vi "Posicionador_VF_Para_Desarrollador.vi"() -> ()   [LabVIEW 2015]
uses:
  <vilib>/Instr/_visa.llb/VISA Configure Serial Port (Instr).vi
panel:
  out "Caracterización Terminada":bool
  in  "Puerto Serial del Gaussmetro":refnum<visa-resource-name>="COM5"
  in  "Ruta de archivo de medición":path=path "C:/Users/PIV/Desktop/Enrico/prueba1.txt"
  out "Medición de campo magnético \nen Teslas [T]":string
  out "?":string="mm"
  out "?":string="mm"
  in  "Listo Y":bool
  in  "Listo X":bool
  in  "Abajo":bool
  in  "Arriba":bool
  in  "Derecha":bool
  in  "Izquierda":bool
  out "Posiciòn en eje X":i32
  out "Posiciòn en eje Y":i32
  in  "Longitud del imán":i32
  in  "Altura del imán":i32
  in  "Puerto Serial de Arduino":refnum<visa-resource-name>="COM12"
  # "Los archivos ejecutables para este programa se encuentran en el repositorio https://github.com/SebRey1995/Posicionador_Caracterizacion.git \n\nPARA LA SECCIÓN DE IDE DE ARDUINO: El archivo denominado \"motor2.ino\" se encuentra en la carpeta denominada \"motor2\". \nPARA LA SECCIÓN DEL EJECUTABLE: El archivo denominado \"Posicionador_VF.exe\" se encuentra en la carpeta \"LabVIEW\".\n\nNota: Para conexión serial entre Gaussmetro y PC, será necesario instalar el archivo ejecutable contenido en la raíz del repositorio proporcionado al principio de este manual. El nombre del archivo es PL2303_64bit_Installer.exe. \nENCENDER GAUSSMETRO MODELO 6010\nIDE DE ARDUINO\n1.  Los pines para la conexión del driver del motor con el Arduino están indicados en el archivo \"motor2.ino\" mediante las variables \"DirPin\", \"StepPin\", \"EnnablePin\" para el motor en X, y \"DirPin2\", \"StepPin2\", \"EnnablePin2\", para el motor en Y. El primer pin refiere a la Dirección; el segundo es el pin para mandarle el tren de pulsos y el tercero para habilitar el motor.\n2.  Para modificar el desplazamiento de 1mm de ambos motores, se deberá modificar el archivo \"motor2.ino\" en la sección después del loop denominada \"void stepMotor\" y \"void Stepmotor2, modificar la variable steps por la cantidad de desplazamiento deseado, tomando en cuenta que steps = 1000 = 1mm de desplazamiento.\n\nAbrir PROGRAMA Posicionador_VF.exe  con los archivos .aliases y .ini en la misma carpeta en la que se ejecuta el archivo  Posicionador_VF.exe \n3.  En el apartado \"Puerto Serial de Arduino\" en la parte superior izquierda, indicar el puerto serial del Arduino. Para verificar en qué puerto se localiza, dirigirse al menú inicio y escribir \"Administrador de dispositivos\". Seguido de esto se dará clic en la opción con el mismo nombre y, en la ventana que emerge, se buscará el apartado \"Puertos COM y LPT\". El puerto del Arduino lleva por nombre inicial \"Arduino\".\n4.  Para seleccionar el puerto del Gaussmetro, dirigirse como en el paso anterior al Administrador de dispositivos y en el apartado Puerto COM y LPT buscar el nombre \"Prolific USB-to-Serial Comm Port\", y el nombre del puerto se especificará entre paréntesis. Este nombre de puerto se especificará en el apartado \"Puerto Serial del Gaussmetro\" ubicado debajo del apartado \"Puerto Serial de Arduino\". \n5.  Ingresar la longitud [en mm] del imán.\n6.  Ingresar la altura [en mm] del imán\n7.  Crear un archivo de texto .txt en la computadora (ubicación a elección) para guardar archivos \n8.  En el apartado \"Ruta de archivo de medición\" se deberá introducir la ubicación del archivo creado en el paso anterior.\n9.  Colocar el imán a caracterizar de forma que la probeta se encuentre del lado superior izquierdo de este. Esto debido a que el movimiento horizontal es hacia la derecha, y el movimiento vertical es hacia abajo.\n10. Verificar Conexión entre el Arduino y el posicionador. Esto se realiza observando un foco led color naranja en la carcasa del motor negro ubicado en el extremo izquierdo del riel horizontal (esto indica que la comunicación serial fue exitosa).\n11.  En caso de estar apagada la luz led naranja del motor, se deberá reiniciar el programa. Para esto se presionará el botón rojo de la parte superior izquierda y se esperará unos segundos hasta ver la luz LED naranja encenderse. Una vez encendida esta luz, se correrá el programa con la flecha blanca de la parte superior izquierda.\n12.  Se deberá iniciar colocando la posición inicial en X (Derecha e Izquierda). Una vez finalizada la posición inicial en X, oprimir el botón \"Listo X\". Al finalizar, deberá parpadear una vez el foco led naranja y se volverá a encender.\n13.  Seguido, se colocará la posición inicial en Y (Arriba y Abajo). Una vez finalizada la posición inicial en Y, oprimir el botón \"Listo Y\". Al finalizar esto, parpadeará una vez el LED naranja y se dará inicio la caracterización deseada.\n\nNOTA: SÓLO PARA LA POSICIÓN DE INICIO EN LA QUE POSICIÓN X = 0 Y POSICIÓN Y = 0, SE TOMARÁ LA MEDICIÓN DE ESE PUNTO, PERO NO SE DESPLAZARÁ 1mm A LA DERECHA. PARA TODOS LOS DEMÁS CASOS SÍ SE DESPLAZARÁ NORMALMENTE.\n\nCreado por:\nSebastian A. Reyes Romero\nContacto: rerosa@ier.unam.mx"
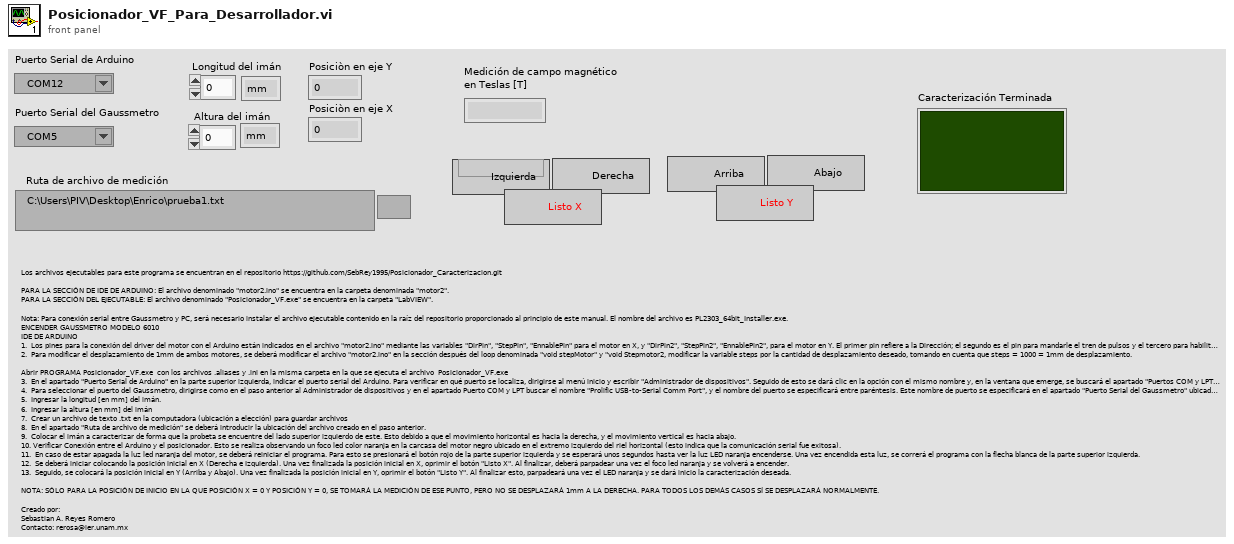
[diagram p1: front panel]
types:
  T1 = enum16{"open", "open or create", "create or replace", "create", "open (read only)"}
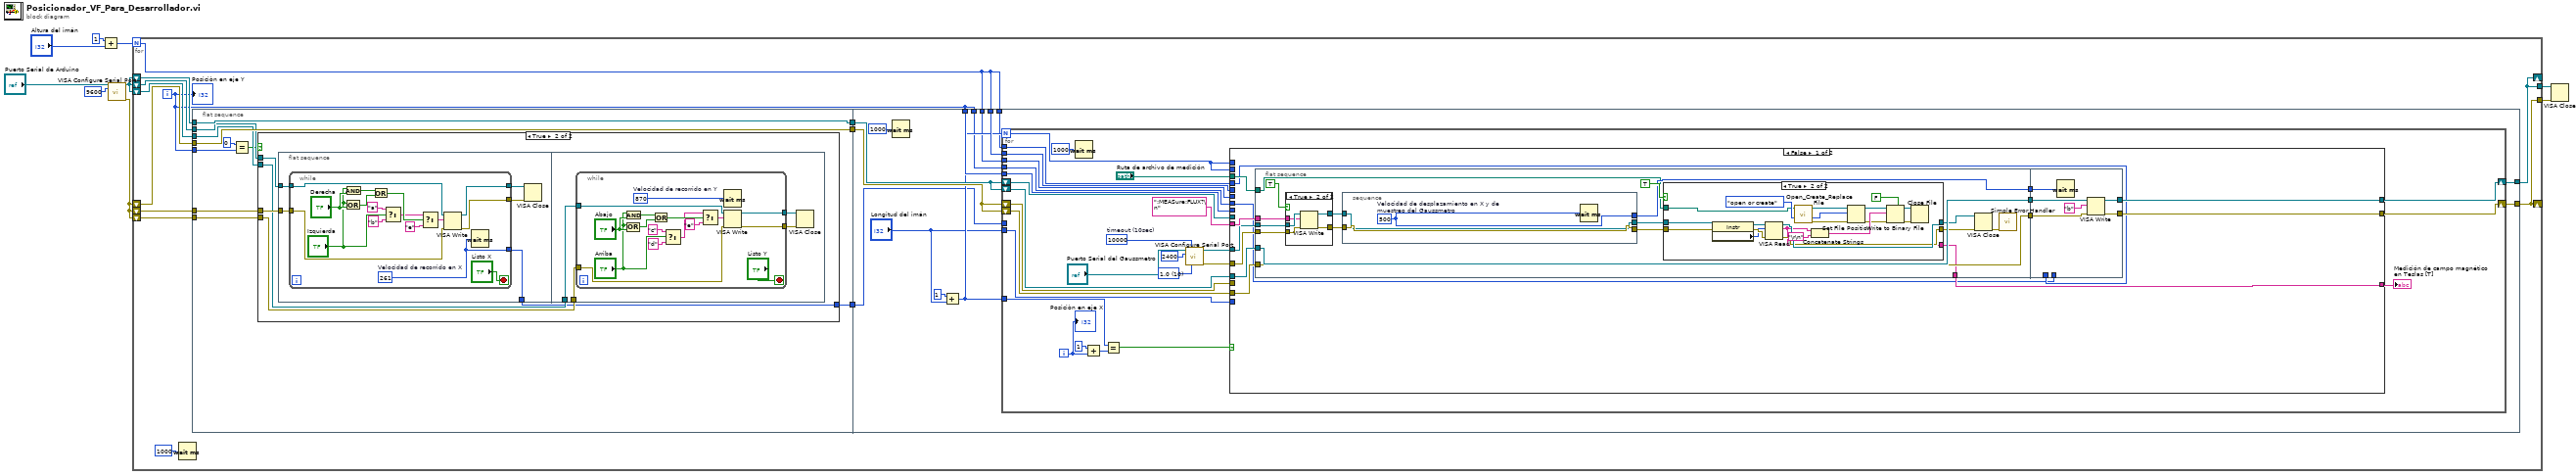
[diagram p0: block diagram]
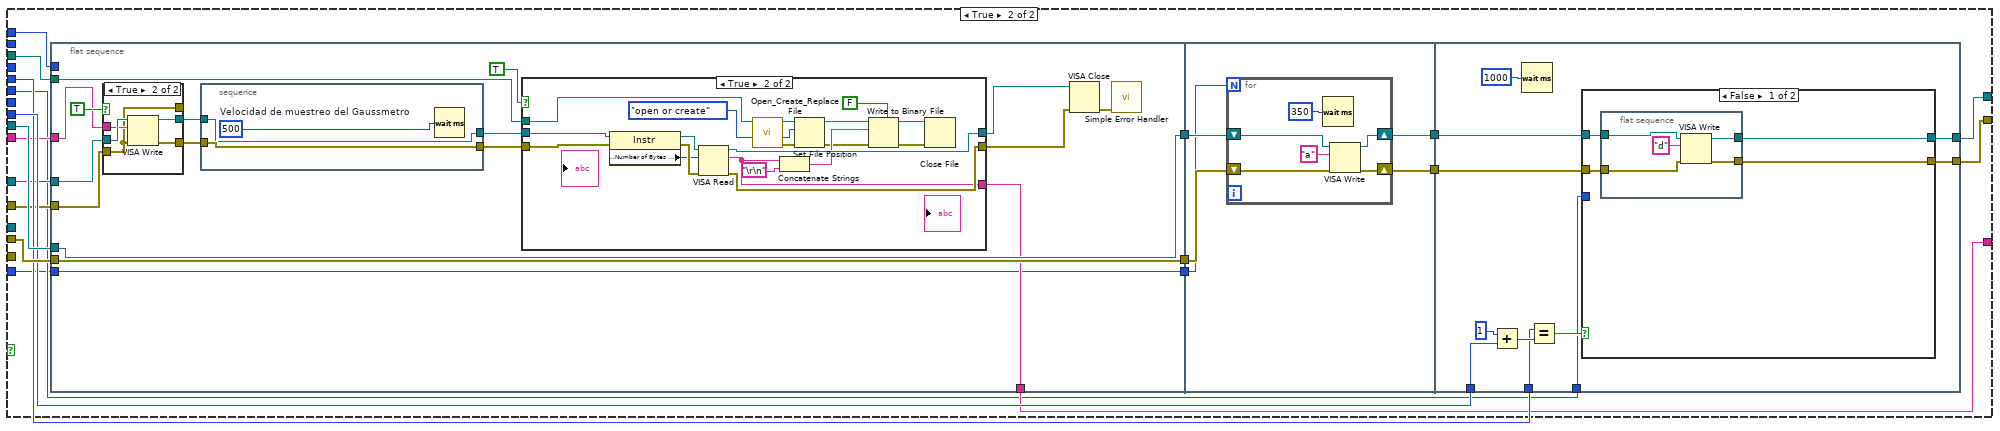
[diagram p5: hidden frame]
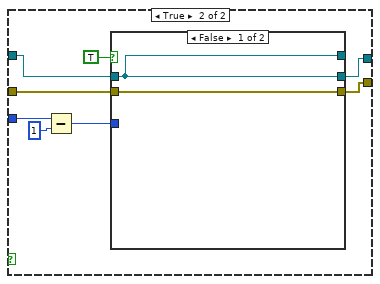
[diagram p8: hidden frame]
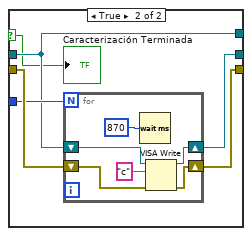
[diagram p9: hidden frame]
diagram:
  n1 = Add(x=1, y="Altura del imán") -> (x+y=w5:i32)
  n2 = call-poly "VISA Configure Serial Port"("VISA resource name"="Puerto Serial de Arduino", "baud rate (9600)"=u32 9600) -> ("VISA resource name out"=w3:refnum<visa-resource-name>, "error out"=w4:errorcluster)  [unwired: 12 in]
  n3 = for {
    N: w5 -> [w11]
    shift-right: [w13] -> _
    shift-right: [w14] -> _
    shift-left: w4 -> [w23]
    shift-left: w3 -> [w19]
    shift-left: w4 -> [w18]
    shift-left: w4 -> [w17]
    shift-left: w3 -> [w15]
    shift-left: w3 -> [w16]
    tunnel: [w14] -> w2
    tunnel: [w13] -> w1
    i -> [w12]
    n4 = Wait (ms)(milliseconds to wait=u32 1000) -> ()  [unwired: 1 out]
    n5 = flat-sequence {
      tunnel: w23 -> [w33]
      tunnel: [w30] -> w21
      tunnel: [w33] -> w20
      tunnel: w19 -> [w29]
      tunnel: w18 -> [w32]
      tunnel: w17 -> [w31]
      tunnel: w16 -> [w30]
      tunnel: w15 -> [w28]
      tunnel: w12 -> [w27]
      tunnel: [w24] -> w10
      tunnel: [w92] -> w14
      tunnel: [w93] -> w13
      tunnel: w12 -> [w89]
      tunnel: w11 -> [w88]
      tunnel: w21 -> [w91]
      tunnel: w20 -> [w90]
      tunnel: w11 -> [w84]
      tunnel: w12 -> [w83]
      tunnel: w11 -> [w82]
      tunnel: w10 -> [w81]
      frame #0 {
        n6 = Equal?(x=0, y=w27) -> (x = y?=w25:bool)
        n7 = case shown="True" w25 {
          tunnel: w32 -> [_ w38]
          tunnel: w31 -> [_ w37]
          tunnel: w29 -> [_ w36]
          tunnel: w28 -> [_ w35]
          tunnel: [_ w34] -> w24
          frame False {
          }
          frame True {
            n8 = flat-sequence {
              tunnel: w35 -> [w43]
              tunnel: w38 -> [w42]
              tunnel: [w39] -> w34
              tunnel: w36 -> [w63]
              tunnel: w37 -> [w62]
              frame #0 {
                n9 = while {
                  tunnel: w43 -> [w50]
                  tunnel: w42 -> [w49]
                  tunnel: [w46] -> w41
                  tunnel: [w45] -> w40
                  tunnel: [w44] -> w39
                  stop <- "Listo X" stop-if-true
                  w44 = u32 261  # Velocidad de recorrido en X
                  n10 = Or(x="Izquierda", y="Derecha") -> (x .or. y?=w56:bool)
                  n11 = And(x="Izquierda", y="Derecha") -> (x .and. y?=w58:bool)
                  n12 = Or(x=w58, y=w56) -> (x .or. y?=w55:bool)
                  n13 = Select(t="a", s="Izquierda", f="b") -> (s? t:f=w48:string)
                  n14 = Select(t=w48, s=w55, f="e") -> (s? t:f=w51:string)
                  n15 = VISA Write(VISA resource name=w50, write buffer=w51, error in (no error)=w49) -> (VISA resource name out=w45:refnum<visa-resource-name>, error out=w46:errorcluster)  [unwired: 1 out]
                  n16 = Wait (ms)(milliseconds to wait=w44) -> ()  [unwired: 1 out]
                }
                n17 = VISA Close(VISA resource name=w40, error in (no error)=w41) -> ()  [unwired: 1 out]
              }
              frame #1 {
                n18 = while {
                  tunnel: w63 -> [w70]
                  tunnel: w62 -> [w69]
                  tunnel: [w65] -> w61
                  tunnel: [w64] -> w60
                  stop <- "Listo Y" stop-if-true
                  w66 = u32 870  # Velocidad de recorrido en Y
                  n19 = Or(x="Arriba", y="Abajo") -> (x .or. y?=w77:bool)
                  n20 = And(x="Arriba", y="Abajo") -> (x .and. y?=w78:bool)
                  n21 = Or(x=w78, y=w77) -> (x .or. y?=w76:bool)
                  n22 = Select(t="c", s="Arriba", f="d") -> (s? t:f=w67:string)
                  n23 = Select(t=w67, s=w76, f="e") -> (s? t:f=w71:string)
                  n24 = Wait (ms)(milliseconds to wait=w66) -> ()  [unwired: 1 out]
                  n25 = VISA Write(VISA resource name=w70, write buffer=w71, error in (no error)=w69) -> (VISA resource name out=w64:refnum<visa-resource-name>, error out=w65:errorcluster)  [unwired: 1 out]
                }
                n26 = VISA Close(VISA resource name=w60, error in (no error)=w61) -> ()  [unwired: 1 out]
              }
            }
          }
        }
      }
      frame #1 {
        n27 = Wait (ms)(milliseconds to wait=u32 1000) -> ()  [unwired: 1 out]
        n28 = Add(x=1, y="Longitud del imán") -> (x+y=w86:i32)
        n29 = for {
          N: w86 -> [w115]
          shift-right: [w118] -> w93
          shift-left: w91 -> [w120]
          shift-right: [w117] -> w92
          shift-left: w90 -> [w119]
          shift-left: w91 -> [w116]
          shift-left: w90 -> [w114]
          tunnel: w86 -> [w110]
          tunnel: w89 -> [w109]
          tunnel: w88 -> [w108]
          tunnel: w84 -> [w97]
          tunnel: w83 -> [w96]
          tunnel: w82 -> [w95]
          tunnel: w81 -> [_]
          tunnel: "Longitud del imán" -> [w94]
          i -> [w113]
          w100 = u16 10 items=["1.0"=10, "1.5"=15, "2.0"=20] ("stop bits (10: 1 bit)")
          w103 = u32 10000  # timeout (10sec)
          n30 = Wait (ms)(milliseconds to wait=u32 1000) -> ()  [unwired: 1 out]
          n31 = Add(x=1, y=w113) -> (x+y=w111:i32)
          n32 = Equal?(x=w110, y=w111) -> (x = y?=w121:bool)
          n33 = call-poly "VISA Configure Serial Port"("VISA resource name"="Puerto Serial del Gaussmetro", "timeout (10sec)"=w103, "baud rate (9600)"=u32 2400, "stop bits (10: 1 bit)"=w100) -> ("VISA resource name out"=w99:refnum<visa-resource-name>, "error out"=w98:errorcluster)  [unwired: 5 in, 5 out]
          n34 = case shown="False" w121 {
            tunnel: w120 -> [_ w209]
            tunnel: w119 -> [_ w208]
            tunnel: [w133 w207] -> w118
            tunnel: [w132 w206] -> w117
            tunnel: w115 -> [_ w205]
            tunnel: w116 -> [w135 _]
            tunnel: w114 -> [w134 _]
            tunnel: w115 -> [_ _]
            tunnel: w109 -> [_ w202]
            tunnel: w108 -> [_ w201]
            tunnel: [w128 w198] -> w106
            tunnel: ":MEASure:FLUX?\n" ("Dato de entrada para\nobtención de flujo magnético 2") -> [w127 w197]
            tunnel: "Ruta de archivo de medición" -> [w126 w196]
            tunnel: w99 -> [w125 w195]
            tunnel: w98 -> [w124 w194]
            tunnel: w97 -> [w123 _]
            tunnel: w96 -> [w122 _]
            tunnel: w95 -> [_ w193]
            tunnel: w94 -> [_ w191]
            frame False {
              n35 = flat-sequence {
                tunnel: w134 -> [w151]
                tunnel: w135 -> [w152]
                tunnel: [w152] -> w131
                tunnel: [w151] -> w130
                tunnel: [w141] -> w129
                tunnel: [w140] -> w128
                tunnel: w127 -> [w139]
                tunnel: w126 -> [w138]
                tunnel: w125 -> [w137]
                tunnel: w124 -> [w136]
                tunnel: [w189] -> w132
                tunnel: [w190] -> w133
                tunnel: w123 -> [_]
                tunnel: w122 -> [_]
                tunnel: w129 -> [w185]
                tunnel: w130 -> [w187]
                tunnel: w131 -> [w188]
                frame #0 {
                  n36 = case shown="True" TRUE ("write") {
                    tunnel: [w157 w162] -> w145
                    tunnel: w137 -> [w156 w161]
                    tunnel: w136 -> [w157 w160]
                    tunnel: [w156 w159] -> w143
                    tunnel: w139 -> [_ w158]
                    frame False {
                    }
                    frame True {
                      n37 = VISA Write(VISA resource name=w161, write buffer=w158, error in (no error)=w160) -> (VISA resource name out=w159:refnum<visa-resource-name>, error out=w162:errorcluster)  [unwired: 1 out]
                    }
                  }
                  n38 = stacked-sequence {
                    tunnel: w145 -> [w155]
                    tunnel: [w155] -> w144
                    tunnel: w143 -> [w154]
                    tunnel: [w154] -> w142
                    tunnel: [w153] -> w141
                    frame #0 {
                      w153 = u32 500  # Velocidad de desplazamiento en X y de muestreo del Gaussmetro
                      n39 = Wait (ms)(milliseconds to wait=w153) -> ()  [unwired: 1 out]
                    }
                  }
                  n40 = case shown="True" TRUE ("read") {
                    tunnel: w144 -> [w164 w181]
                    tunnel: [w164 w178] -> w149
                    tunnel: [w163 w184] -> w148
                    tunnel: w142 -> [w163 w183]
                    tunnel: [_ w166] -> w140
                    tunnel: w138 -> [_ w165]
                    frame False {
                    }
                    frame True {
                      n41 = property class="Instr"(reference=w183, error in=w181) -> (reference out=w182:refnum<visa-resource-name>, error out=w180:errorcluster, "Serial Settings:Number of Bytes at Serial Port"=w179:u32)
                      n42 = VISA Read(VISA resource name=w182, byte count=w179, error in (no error)=w180) -> (VISA resource name out=w184:refnum<visa-resource-name>, read buffer=w166:string, error out=w178:errorcluster)  [unwired: 1 out]
                      n43 = call <vilib>:"Open_Create_Replace File.vi"("function (open:0)"=T1."open or create", "file path"=w165) -> ("error out"=w176:errorcluster, "file size (bytes)"=w174:i32, "refnum"=w175:refnum<file>)  [unwired: 6 in, 1 out]
                      n44 = Concatenate Strings(w166, "\r\n") -> (w170:string)
                      n45 = Set File Position(offset (in bytes) (0)=w174, refnum=w175, error in=w176) -> (refnum out=w169:refnum<file>, error out=w168:errorcluster)  [unwired: 1 in]
                      n46 = Write to Binary File(file (use dialog)=w169, data=w170, error in=w168, 5:FALSE ("prepend array or string size? (T)")) -> (refnum out=w172:refnum<file>, error out=w173:errorcluster)  [unwired: 2 in, 1 out]
                      n47 = Close File(refnum=w172, error in=w173) -> ()  [unwired: 2 out]
                    }
                  }
                  n48 = VISA Close(VISA resource name=w148, error in (no error)=w149) -> (error out=w147:errorcluster)
                  n49 = call <vilib>:"Simple Error Handler.vi"("error in (no error)"=w147) -> ()  [unwired: 1 in, 8 out]
                }
                frame #1 {
                  n50 = Wait (ms)(milliseconds to wait=w185) -> ()  [unwired: 1 out]
                  n51 = VISA Write(VISA resource name=w188, write buffer="b", error in (no error)=w187) -> (VISA resource name out=w190:refnum<visa-resource-name>, error out=w189:errorcluster)  [unwired: 1 out]
                }
              }
            }
            frame True {
              n52 = flat-sequence {
                tunnel: w205 -> [_]
                tunnel: w208 -> [w225]
                tunnel: w209 -> [w226]
                tunnel: [w226] -> w200
                tunnel: [w225] -> w199
                tunnel: [w215] -> w198
                tunnel: w197 -> [w214]
                tunnel: w196 -> [w213]
                tunnel: w195 -> [w212]
                tunnel: w194 -> [w211]
                tunnel: [w210] -> w192
                tunnel: w191 -> [w210]
                tunnel: [w261] -> w204
                tunnel: [w260] -> w203
                tunnel: w200 -> [w263]
                tunnel: w199 -> [w262]
                tunnel: w192 -> [w259]
                tunnel: [w279] -> w206
                tunnel: [w280] -> w207
                tunnel: w201 -> [w273]
                tunnel: w202 -> [w276]
                tunnel: w203 -> [w277]
                tunnel: w204 -> [w278]
                tunnel: w193 -> [w270]
                frame #0 {
                  n53 = case shown="True" TRUE ("write 2") {
                    tunnel: [w230 w236] -> w219
                    tunnel: w212 -> [w231 w235]
                    tunnel: [w230 w232] -> _
                    tunnel: [w231 w234] -> w217
                    tunnel: w214 -> [_ w233]
                    tunnel: w211 -> [w230 w232]
                    frame False {
                    }
                    frame True {
                      n54 = VISA Write(VISA resource name=w235, write buffer=w233, error in (no error)=w232) -> (VISA resource name out=w234:refnum<visa-resource-name>, error out=w236:errorcluster)  [unwired: 1 out]
                    }
                  }
                  n55 = stacked-sequence {
                    tunnel: w219 -> [w229]
                    tunnel: [w229] -> w218
                    tunnel: w217 -> [w228]
                    tunnel: [w228] -> w216
                    frame #0 {
                      w227 = u32 500  # Velocidad de muestreo del Gaussmetro
                      n56 = Wait (ms)(milliseconds to wait=w227) -> ()  [unwired: 1 out]
                    }
                  }
                  n57 = case shown="True" TRUE ("read 2") {
                    tunnel: w218 -> [w238 w255]
                    tunnel: [w238 w252] -> w223
                    tunnel: [w237 w258] -> w222
                    tunnel: w216 -> [w237 w257]
                    tunnel: [_ w240] -> w215
                    tunnel: w213 -> [_ w239]
                    frame False {
                    }
                    frame True {
                      n58 = property class="Instr"(reference=w257, error in=w255) -> (reference out=w256:refnum<visa-resource-name>, error out=w254:errorcluster, "Serial Settings:Number of Bytes at Serial Port"=w253:u32)
                      n59 = VISA Read(VISA resource name=w256, byte count=w253, error in (no error)=w254) -> (VISA resource name out=w258:refnum<visa-resource-name>, read buffer=w240:string, error out=w252:errorcluster)  [unwired: 1 out]
                      n60 = call <vilib>:"Open_Create_Replace File.vi"("function (open:0)"=T1."open or create", "file path"=w239) -> ("error out"=w250:errorcluster, "file size (bytes)"=w248:i32, "refnum"=w249:refnum<file>)  [unwired: 6 in, 1 out]
                      n61 = Concatenate Strings(w240, "\r\n") -> (w244:string)
                      n62 = Set File Position(offset (in bytes) (0)=w248, refnum=w249, error in=w250) -> (refnum out=w243:refnum<file>, error out=w242:errorcluster)  [unwired: 1 in]
                      n63 = Write to Binary File(file (use dialog)=w243, data=w244, error in=w242, 5:FALSE ("prepend array or string size? (T)")) -> (refnum out=w246:refnum<file>, error out=w247:errorcluster)  [unwired: 2 in, 1 out]
                      n64 = Close File(refnum=w246, error in=w247) -> ()  [unwired: 2 out]
                    }
                  }
                  n65 = VISA Close(VISA resource name=w222, error in (no error)=w223) -> (error out=w221:errorcluster)
                  n66 = call <vilib>:"Simple Error Handler.vi"("error in (no error)"=w221) -> ()  [unwired: 1 in, 8 out]
                }
                frame #1 {
                  n67 = for {
                    N: w259 -> [_]
                    shift-right: [w267] -> w261
                    shift-left: w263 -> [w269]
                    shift-right: [w266] -> w260
                    shift-left: w262 -> [w268]
                    n68 = Wait (ms)(milliseconds to wait=u32 350) -> ()  [unwired: 1 out]
                    n69 = VISA Write(VISA resource name=w269, write buffer="a", error in (no error)=w268) -> (VISA resource name out=w267:refnum<visa-resource-name>, error out=w266:errorcluster)  [unwired: 1 out]
                  }
                }
                frame #2 {
                  n70 = Add(x=1, y=w276) -> (x+y=w274:i32)
                  n71 = Wait (ms)(milliseconds to wait=u32 1000) -> ()  [unwired: 1 out]
                  n72 = Equal?(x=w273, y=w274) -> (x = y?=w272:bool)
                  n73 = case shown="False" w272 {
                    tunnel: w278 -> [w284 w297]
                    tunnel: [w283 w295] -> w280
                    tunnel: w277 -> [w282 w296]
                    tunnel: [w281 w294] -> w279
                    tunnel: w270 -> [_ w292]
                    frame False {
                      n74 = flat-sequence {
                        tunnel: [w288] -> w281
                        tunnel: [w289] -> w283
                        tunnel: w282 -> [w286]
                        tunnel: w284 -> [w287]
                        frame #0 {
                          n75 = VISA Write(VISA resource name=w287, write buffer="d", error in (no error)=w286) -> (VISA resource name out=w289:refnum<visa-resource-name>, error out=w288:errorcluster)  [unwired: 1 out]
                        }
                      }
                    }
                    frame True {
                      n76 = Subtract(x=w292, y=1) -> (x-y=w290:i32)
                      n77 = case shown="False" TRUE {
                        selector: TRUE -> [_ w300]
                        tunnel: [w298 w301] -> _
                        tunnel: w296 -> [w299 w305]
                        tunnel: [w298 w304] -> w295
                        tunnel: [w299 w303] -> w294
                        tunnel: w290 -> [_ w302]
                        tunnel: w297 -> [w298 w301]
                        frame False {
                        }
                        frame True {
                          n78 = for {
                            N: w302 -> [_]
                            shift-right: [w309] -> w304
                            shift-left: w301 -> [w311]
                            shift-right: [w308] -> w303
                            shift-left: w305 -> [w310]
                            n79 = Wait (ms)(milliseconds to wait=u32 870) -> ()  [unwired: 1 out]
                            n80 = VISA Write(VISA resource name=w311, write buffer="c", error in (no error)=w310) -> (VISA resource name out=w309:refnum<visa-resource-name>, error out=w308:errorcluster)  [unwired: 1 out]
                          }
                          "Caracterización Terminada" <- w300
                        }
                      }
                    }
                  }
                }
              }
            }
          }
          "Medición de campo magnético \nen Teslas [T]" <- w106
          "Posiciòn en eje X" <- w113
        }
      }
    }
    "Posiciòn en eje Y" <- w12
  }
  n81 = VISA Close(VISA resource name=w1, error in (no error)=w2) -> ()  [unwired: 1 out]
